vi "PQport.vi"(7 "error in (no error)":errorcluster, 10 "conn":u32) -> (0 "error out":errorcluster, 2 "port":string, 3 "conn_out":u32)   [LabVIEW 2019, in "libpqlv.lvlib"]
doc: "Returns the port of the connection."
uses:
  libpqlv.lvlib
  libpq.dll
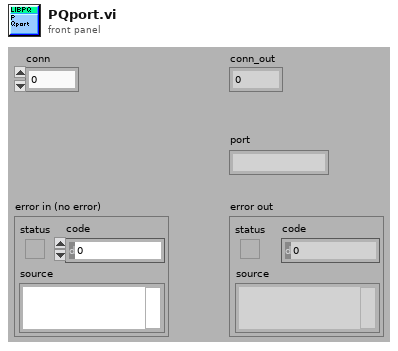
[diagram p1: front panel]
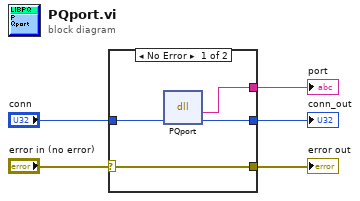
[diagram p0: block diagram]
diagram:
  n1 = case shown="No Error" "error in (no error)" {
    selector: "error in (no error)" -> [w9 w11]
    tunnel: [w9 w11] -> w4
    tunnel: [w8 _] -> w3
    tunnel: "conn" -> [w7 w10]
    tunnel: [w6 w10] -> w1
    frame No Error {
      n2 = dll-call lib="libpq.*" fn="PQport"("conn"=w7) -> ("port"=w8:string, "conn"=w6:u32)  [unwired: 3 in, 2 out]
    }
    frame Error {
    }
  }
  "port" <- w3
  "error out" <- w4
  "conn_out" <- w1
